vi "PlayerStop.vi"(11 "NXT":T1={"Hardware"="NXT", "Flattened String"=""}) -> (3 "NXT":T1={"Hardware"="NXT", "Flattened String"=""})   [LabVIEW 2010, in "Player.lvlib"]
uses:
  Player.lvlib
  <vilib>/NXT/Subs/LVHSConnector.ctl
  CLIB/CThread/XNodes/referencenode/CThread VI Reference.xnode
  CLIB/CThread/XNodes/terminalnode/CThread VI Terminal Node.xnode
  CLIB/CThread/Base/CThread Base - VI Reference.vi
  CLIB/CThread/Base/CThread Base - Cancel.vi
  PlayerMain.vi
  CLIB/CThread/CThread.lvlib
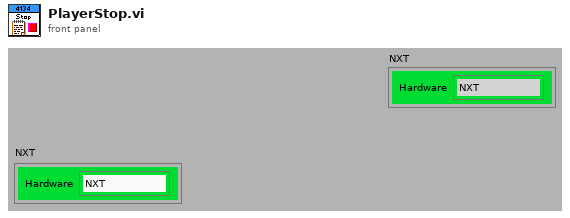
[diagram p1: front panel]
types:
  T1 = typedef "LVHSConnector.ctl" = cluster{"Hardware":string, "Flattened String":string}
  T2 = typedef "NXT_FileStatusCodes.ctl" = u16
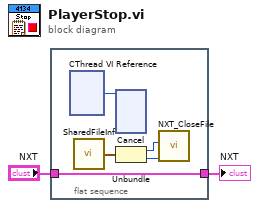
[diagram p0: block diagram]
diagram:
  n1 = flat-sequence {
    tunnel: "NXT" -> [w6]
    tunnel: [w6] -> w2
    frame #0 {
      n2 = xnode "CThread VI Reference"() -> ("PlayerMain.vi"=w7:i32)
      n3 = call "SharedFileInf.vi"() -> ("FileInf"=w5:cluster{"Error in":T2, "File Handle in":u8})  [unwired: 2 in]
      n4 = xnode "Cancel"("CLIB VI Reference"=w7) -> ()  [unwired: 1 out]
      n5 = Unbundle(w5) -> ("Error in"=w4:T2, "File Handle in"=w3:u8)
      n6 = call <vilib>:"NXT_CloseFile.vi"("Error in"=w3, "File Handle"=w4) -> ()  [unwired: 8 in, 2 out]
    }
  }
  "NXT" <- w2
